vi "Bootloader - Open Communication (COM).vi"(0 "COM Port":refnum<visa-resource-name>="COMx", 11 "error in (no error)":errorcluster) -> (4 "COM Port":refnum<visa-resource-name>, 15 "error out":errorcluster)   [LabVIEW 2010]
uses:
  <vilib>/Instr/_visa.llb/VISA Configure Serial Port (Instr).vi
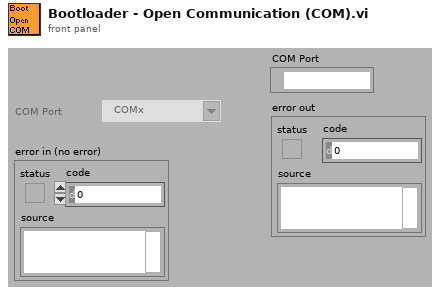
[diagram p1: front panel]
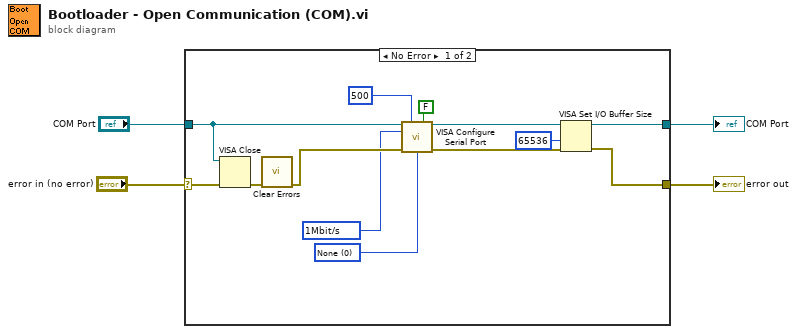
[diagram p0: block diagram]
diagram:
  n1 = case shown="No Error" "error in (no error)" {
    selector: "error in (no error)" -> [w5 w18]
    tunnel: "COM Port" -> [w11 w19]
    tunnel: [w8 w18] -> w3
    tunnel: [w7 w19] -> w1
    frame No Error {
      w12 = u32 1000000 items=["250Kbit/s"=250000, "500kbit/s"=500000, "1Mbit/s"=1000000, "2Mbit/s"=2000000, "4Mbit/s"=4000000] ("baud rate")
      w13 = u16 0 items=["None", "XON/XOFF", "RTS/CTS", "XON/XOFF & RTS/CTS", "DTR/DSR", "XON/XOFF & DTR/DSR"] ("flow control (0:none)")
      n2 = VISA Close(VISA resource name=w11, error in (no error)=w5) -> (error out=w14:errorcluster)
      n3 = call <vilib>:"Clear Errors.vi"("error in (no error)"=w14) -> ("error out"=w16:errorcluster)  [unwired: 6 in]
      n4 = call-poly "VISA Configure Serial Port"("VISA resource name"=w11, "timeout (10sec)"=u32 500, "Enable Termination\nChar (T)"=FALSE ("Enable Termination\nChar (T)"), "baud rate (9600)"=w12, "error in (no error)"=w16, "flow control (0:none)"=w13) -> ("VISA resource name out"=w9:refnum<visa-resource-name>, "error out"=w10:errorcluster)  [unwired: 8 in]
      n5 = VISA Set I/O Buffer Size(VISA resource name=w9, size (4096)=u32 65536, error in (no error)=w10) -> (VISA resource name out=w7:refnum<visa-resource-name>, error out=w8:errorcluster)  [unwired: 1 in]
    }
    frame Error {
    }
  }
  "error out" <- w3
  "COM Port" <- w1
